vi "StressDist_report.vi"(5 "Corrigido":bool, 7 "StressDist_types":T1, 8 "Error In":errorcluster, 11 "main_FGV_data":T2={"pipe_properties"={"out_radius"=0.0, "in_radius"=0.0, "out_diameter"=0.0, "in_diameter"=0.0, "thickness"=0.0, "inertia"=0.0, "area"=0.0}, "DirPath"=path "L:/Documentos/00 SERVIÇOS/Tensão residual/Olapa 10-2017/Dados/Primeira Seção/Furos", "DirReport"=path "L:/Documentos/00 SERVIÇOS/Tensão residual/Olapa 10-2017/RelatóriosOlapa/Teste", "Points"=[], "ovalization_data"={"AngOval"=[0.0, 60.0, 120.0, 22.5, 45.0, 67.5, 90.0, 112.5, 135.0, 157.5, 180.0], "OvalDiam"=[324.25, 324.6, 324.55, 324.25, 324.55, 324.65, 324.6, 324.65, 324.55, 324.5, 324.4], "Plots"={"Ref"={"X"=[], "Y"=[]}, "Elipse"={"X"=[], "Y"=[]}, "Points"={"X"=[], "Y"=[]}}, "Ampliation"=100.0, "Results"={"MD"=0.0, "mD"=0.0, "Dmed"=0.0, "Oval"=0.0, "ang"=0.0, "X0"=0.0, "Y0"=0.0}, "fit"=[]}, "StressDist_data"={"Long"={"Plot"=[], "Fit"=[], "ColorMap"=[], "Data"=[], "peirce_data"={"Plot"=[], "Index removidos"=[]}}, "Circ"={"Plot"=[], "Fit"=[], "ColorMap"=[], "Data"=[], "peirce_data"={"Plot"=[], "Index removidos"=[]}}, "Shear"={"Plot"=[], "Fit"=[], "ColorMap"=[], "Data"=[], "peirce_data"={"Plot"=[], "Index removidos"=[]}}, "Equivalent"={"Plot"=[], "Fit"=[], "ColorMap"=[], "Data"=[], "peirce_data"={"Plot"=[], "Index removidos"=[]}}}, "pressure_data"={"Pressure"=[], "StressCircOval"=[], "StressCirc"=[], "StressLong"=[], "Plot"=[], "Angle"=[]}, "Reload"=FALSE}) -> (0 "Error Out":errorcluster, 3 "main_FGV_data-out":T2={"pipe_properties"={"out_radius"=0.0, "in_radius"=0.0, "out_diameter"=0.0, "in_diameter"=0.0, "thickness"=0.0, "inertia"=0.0, "area"=0.0}, "DirPath"=path "L:/Documentos/00 SERVIÇOS/Tensão residual/Olapa 10-2017/Dados/Primeira Seção/Furos", "DirReport"=path "L:/Documentos/00 SERVIÇOS/Tensão residual/Olapa 10-2017/RelatóriosOlapa/Teste", "Points"=[], "ovalization_data"={"AngOval"=[0.0, 60.0, 120.0, 22.5, 45.0, 67.5, 90.0, 112.5, 135.0, 157.5, 180.0], "OvalDiam"=[324.25, 324.6, 324.55, 324.25, 324.55, 324.65, 324.6, 324.65, 324.55, 324.5, 324.4], "Plots"={"Ref"={"X"=[], "Y"=[]}, "Elipse"={"X"=[], "Y"=[]}, "Points"={"X"=[], "Y"=[]}}, "Ampliation"=100.0, "Results"={"MD"=0.0, "mD"=0.0, "Dmed"=0.0, "Oval"=0.0, "ang"=0.0, "X0"=0.0, "Y0"=0.0}, "fit"=[]}, "StressDist_data"={"Long"={"Plot"=[], "Fit"=[], "ColorMap"=[], "Data"=[], "peirce_data"={"Plot"=[], "Index removidos"=[]}}, "Circ"={"Plot"=[], "Fit"=[], "ColorMap"=[], "Data"=[], "peirce_data"={"Plot"=[], "Index removidos"=[]}}, "Shear"={"Plot"=[], "Fit"=[], "ColorMap"=[], "Data"=[], "peirce_data"={"Plot"=[], "Index removidos"=[]}}, "Equivalent"={"Plot"=[], "Fit"=[], "ColorMap"=[], "Data"=[], "peirce_data"={"Plot"=[], "Index removidos"=[]}}}, "pressure_data"={"Pressure"=[], "StressCircOval"=[], "StressCirc"=[], "StressLong"=[], "Plot"=[], "Angle"=[]}, "Reload"=FALSE})   [LabVIEW 2016]
uses:
  MainFGV/main_FGV_data.ctl
  MainFGV/pipe_properties.ctl
  StressCalculations/point_data.ctl
  Ovalization/ovalization_data.ctl
  StressDist_data.ctl
  StressDist_single_data.ctl
  Peirce/peirce_data.ctl
  Pressure/pressure_data.ctl
  StressDist_types.ctl
  Report/report_mods.ctl
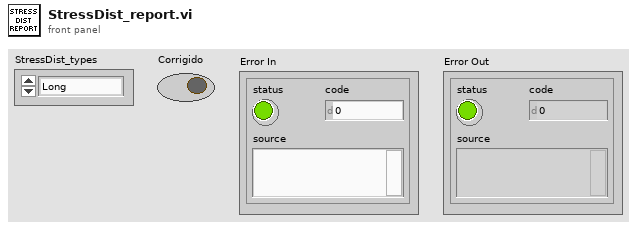
[diagram p1: front panel]
types:
  T1 = typedef "StressDist_types.ctl" = enum16{"Long", "Circ", "Shear", "Equivalent"}
  T2 = typedef "main_FGV_data.ctl" = cluster{"pipe_properties":T3, "DirPath":path, "DirReport":path, "Points":T4[], "ovalization_data":T5, "StressDist_data":T6, "pressure_data":T9, "Reload":bool}
  T3 = typedef "pipe_properties.ctl" = cluster{"out_radius":dbl, "in_radius":dbl, "out_diameter":dbl, "in_diameter":dbl, "thickness":dbl, "inertia":dbl, "area":dbl}
  T4 = typedef "point_data.ctl" = cluster{"LongStress":dbl, "CircStress":dbl, "ShearStress":dbl, "Pressure":dbl, "Angle":dbl, "Thickness":dbl, "HoleDiam":dbl, "EquiStress":dbl, "S1":dbl, "S2":dbl, "Beta":dbl}
  T5 = typedef "ovalization_data.ctl" = cluster{"AngOval":dbl[], "OvalDiam":dbl[], "Plots":cluster{"Ref":cluster{"X":dbl[], "Y":dbl[]}, "Elipse":cluster{"X":dbl[], "Y":dbl[]}, "Points":cluster{"X":dbl[], "Y":dbl[]}}, "Ampliation":dbl, "Results":cluster{"MD":dbl, "mD":dbl, "Dmed":dbl, "Oval":dbl, "ang":dbl, "X0":dbl, "Y0":dbl}, "fit":dbl[]}
  T6 = typedef "StressDist_data.ctl" = cluster{"Long":T7, "Circ":T7, "Shear":T7, "Equivalent":T7}
  T7 = typedef "StressDist_single_data.ctl" = cluster{"Plot":cluster{"Angle":dbl[], "Stress":dbl[]}[], "Fit":dbl[], "ColorMap":dbl[][], "Data":string[][], "peirce_data":T8}
  T8 = typedef "peirce_data.ctl" = cluster{"Plot":cluster{"Array":dbl[], "Array":dbl[]}[], "Index removidos":i32[]}
  T9 = typedef "pressure_data.ctl" = cluster{"Pressure":dbl[], "StressCircOval":dbl[], "StressCirc":dbl[], "StressLong":dbl[], "Plot":cluster{"Angle":dbl[], "Stress":dbl[]}[], "Angle":dbl[]}
  T10 = typedef "report_mods.ctl" = enum16{"Init", "Table", "Graph", "TablefromGraph", "End"}
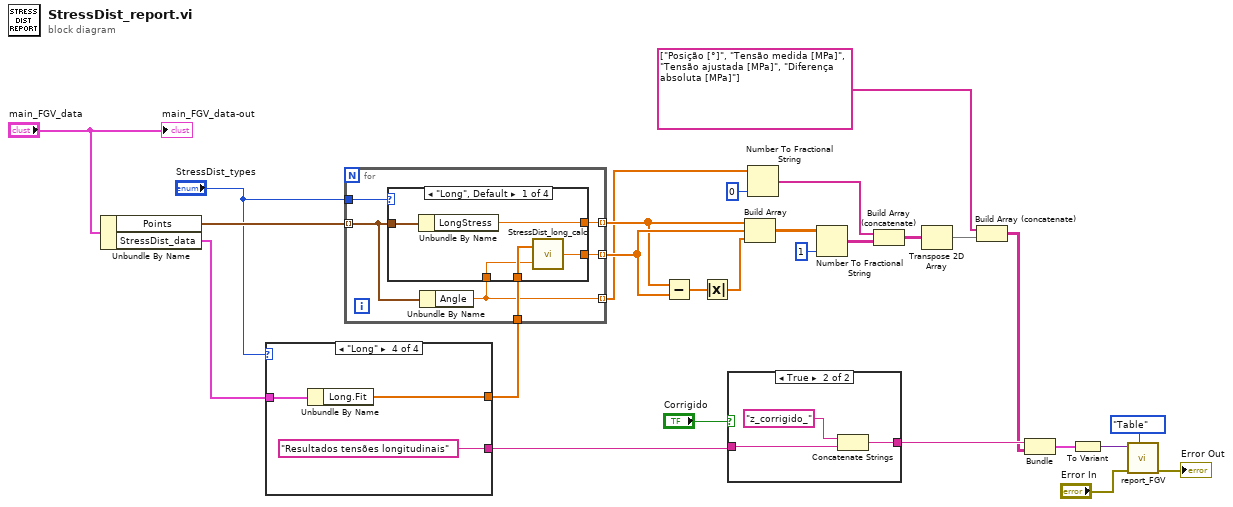
[diagram p0: block diagram]
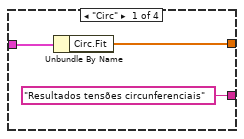
[diagram p2: hidden frame]
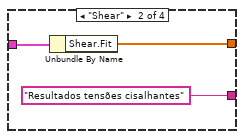
[diagram p3: hidden frame]
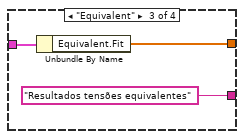
[diagram p4: hidden frame]
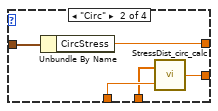
[diagram p5: hidden frame]
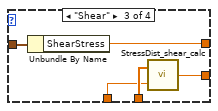
[diagram p6: hidden frame]
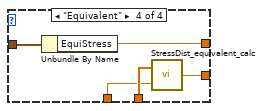
[diagram p7: hidden frame]
diagram:
  n1 = Unbundle By Name("main_FGV_data") -> ("Points"=w19:T4[], "StressDist_data"=w17:T6)
  n2 = case shown="\"Long\"" "StressDist_types" {
    tunnel: w17 -> [w30 w33 w36 w39]
    tunnel: [w29 w32 w35 w38] -> w15
    tunnel: ["Resultados tensões circunferenciais" "Resultados tensões cisalhantes" "Resultados tensões equivalentes" "Resultados tensões longitudinais"] -> w16
    frame "Circ" {
      n3 = Unbundle By Name(w30) -> ("Circ.Fit"=w29:dbl[])
    }
    frame "Shear" {
      n4 = Unbundle By Name(w33) -> ("Shear.Fit"=w32:dbl[])
    }
    frame "Equivalent" {
      n5 = Unbundle By Name(w36) -> ("Equivalent.Fit"=w35:dbl[])
    }
    frame "Long" {
      n6 = Unbundle By Name(w39) -> ("Long.Fit"=w38:dbl[])
    }
  }
  n7 = for {
    tunnel: "StressDist_types" -> [w45]
    tunnel: w19 -> [w44] mode=indexing
    tunnel: [w43] -> w11 mode=indexing
    tunnel: w15 -> [w42]
    tunnel: [w41] -> w12 mode=indexing
    tunnel: [w40] -> w6 mode=indexing
    n8 = Unbundle By Name(w44) -> ("Angle"=w40:dbl)
    n9 = case shown="\"Long\", Default" w45 {
      tunnel: w44 -> [w50 w55 w60 w65]
      tunnel: [w49 w54 w59 w64] -> w43
      tunnel: w40 -> [w46 w53 w56 w61]
      tunnel: w42 -> [w47 w52 w58 w62]
      tunnel: [w48 w51 w57 w63] -> w41
      frame "Long", Default {
        n10 = Unbundle By Name(w50) -> ("LongStress"=w49:dbl)
        n11 = call "StressDist_long_calc.vi"("Angle"=w46, "Parameters"=w47) -> ("Stress"=w48:dbl)
      }
      frame "Circ" {
        n12 = Unbundle By Name(w55) -> ("CircStress"=w54:dbl)
        n13 = call "StressDist_circ_calc.vi"("Angle"=w53, "Parameters"=w52) -> ("Stress"=w51:dbl)
      }
      frame "Shear" {
        n14 = Unbundle By Name(w60) -> ("ShearStress"=w59:dbl)
        n15 = call "StressDist_shear_calc.vi"("Angle"=w56, "Parameters"=w58) -> ("Stress"=w57:dbl)
      }
      frame "Equivalent" {
        n16 = Unbundle By Name(w65) -> ("EquiStress"=w64:dbl)
        n17 = call "StressDist_equivalent_calc.vi"("Angle"=w61, "Parameters"=w62) -> ("Stress"=w63:dbl)  [unwired: 1 in]
      }
    }
  }
  n18 = Subtract(x=w11, y=w12) -> (x-y=w14:dbl[])
  n19 = Absolute Value(x=w14) -> (abs(x)=w13:dbl[])
  n20 = case shown="True" "Corrigido" {
    tunnel: w16 -> [w66 w69]
    tunnel: [w66 w68] -> w21
    frame False {
    }
    frame True {
      n21 = Concatenate Strings("z_corrigido_" ("string"), w69) -> (w68:string)
    }
  }
  n22 = Build Array(w11, w12, w13) -> (w5:dbl[][])
  n23 = Number To Fractional String(number=w6, precision (6)=i16 0) -> (F-format string=w3:string[])  [unwired: 2 in]
  n24 = Number To Fractional String(number=w5, precision (6)=i16 1) -> (F-format string=w4:string[][])  [unwired: 2 in]
  n25 = Build Array (concatenate)(w3, w4) -> (w2:string[][])
  n26 = Transpose 2D Array(2D array=w2) -> (transposed array=w1:string[][])
  n27 = Build Array (concatenate)(string[] ["Posição [°]", "Tensão medida [MPa]", "Tensão ajustada [MPa]", "Diferença absoluta [MPa]"] ("element"), w1) -> (w8:string[][])
  n28 = Bundle(w21, w8) -> (w26:cluster{string, string[][]})  [unwired: 1 in]
  n29 = To Variant(anything=w26) -> (Variant=w25:variant)
  n30 = call "report_FGV.vi"("report_mods"=report_mods."Table", "Error In"="Error In", "Data in"=w25) -> ("Error Out"=→"Error Out":errorcluster)  [unwired: 8 in]
  "main_FGV_data-out" <- "main_FGV_data"
